vi "Duplicate.vi"(8 "error in":errorcluster, 10 "parameters":variant, 11 "group in":refnum<class "Group.lvclass">) -> (0 "error out":errorcluster, 3 "group copy":refnum<class "Group.lvclass">)   [LabVIEW 2015, in "Group.lvclass"]
doc: "Copyright 2017 National Instruments Corporation\n\nLicensed under the Apache License, Version 2.0 (the \"License\"); you may not use this file except in compliance with the License. You may obtain a copy of the License at http://www.apache.org/licenses/LICENSE-2.0\nUnless required by applicable law or agreed to in writing, software distributed under the License is distributed on an \"AS IS\" BASIS, WITHOUT WARRANTIES OR CONDITIONS OF ANY KIND, either express or implied. See the License for the specific language governing permissions and limitations under the License."
uses:
  Group.lvclass
  Group.lvclass/Group.ctl
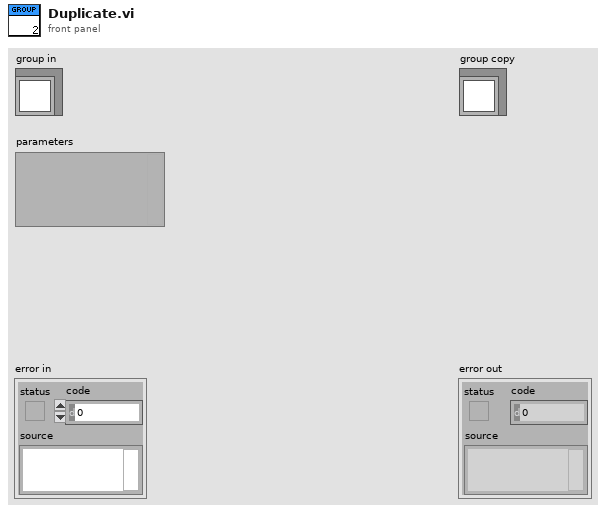
[diagram p1: front panel]
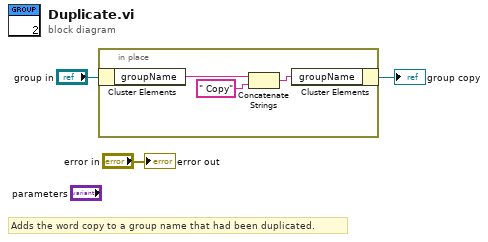
[diagram p0: block diagram]
diagram:
  # "Adds the word copy to a group name that had been duplicated."
  n1 = in-place {
    n2 = in-place-cluster #1("group in") -> ("groupName"=w6:string)
    n3 = Concatenate Strings(w6, " Copy" ("string")) -> (w4:string)
    n4 = in-place-cluster #1("groupName"=w4) -> (→"group copy":refnum<class "Group.lvclass">)
  }
  "error out" <- "error in"
